vi "FGV_Counter_Boolean.vi"(7 "Reset (T)/Count (F)":bool, 8 "error in (no error)":errorcluster, 11 "Time Limit (10)":dbl=10.0) -> (0 "error out":errorcluster, 2 "Time Elapsed?":bool, 3 "Time":dbl)   [LabVIEW 2020]
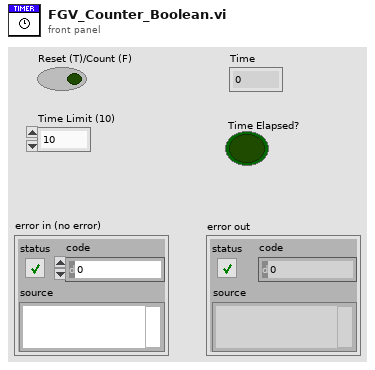
[diagram p1: front panel]
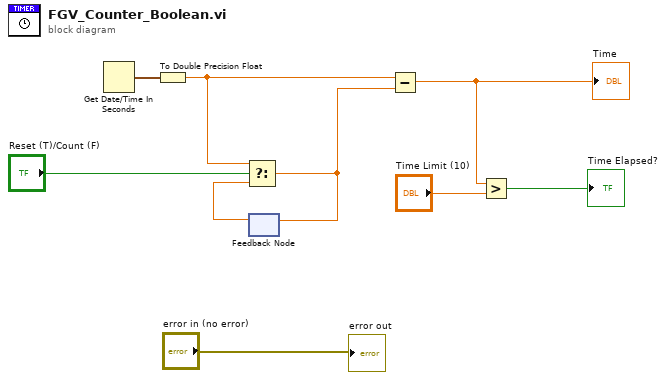
[diagram p0: block diagram]
diagram:
  n1 = Get Date/Time In Seconds() -> (seconds since 1Jan1904=w4:timestamp)
  n2 = To Double Precision Float(number=w4) -> (double precision float=w5:dbl)
  n3 = feedback #1() -> (w6:dbl)  [unwired: 1 in]
  n4 = Select(t=w5, s="Reset (T)/Count (F)", f=w6) -> (s? t:f=w7:dbl)
  n5 = feedback-in #1(w7) -> ()
  n6 = Subtract(x=w5, y=w7) -> (x-y=w1:dbl)
  "Time" <- w1
  n7 = Greater?(x=w1, y="Time Limit (10)") -> (0:→"Time Elapsed?":bool)
  "error out" <- "error in (no error)"
